vi "write_to_Sumitomo_F70.vi"(0 "VISA resource name":refnum<visa-resource-name>, 2 "Write String":string="$", 11 "error in (no error)":errorcluster) -> (4 "VISA resource name out":refnum<visa-resource-name>, 13 "Written String":string, 15 "error out":errorcluster)   [LabVIEW 2023]
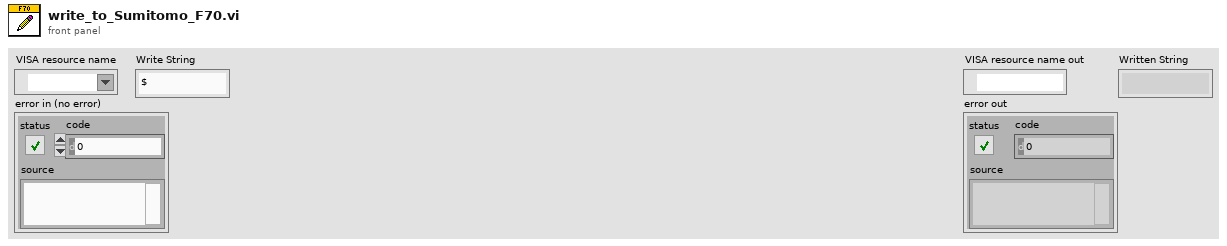
[diagram p1: front panel]
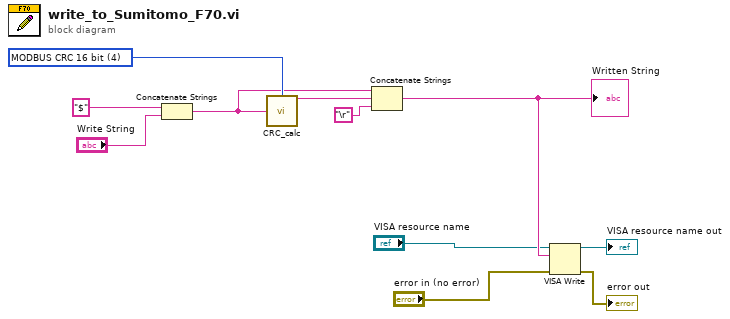
[diagram p0: block diagram]
diagram:
  w9 = u32 4 items=["XOR", "8 bit sum (MOD 100h)", "8 bit LRC", "16 bit sum (MOD 10000h)", "MODBUS CRC 16 bit", "XOR 16 bit"] ("Type (0)")
  n1 = Concatenate Strings("$", "Write String") -> (w8:string)
  n2 = call "CRC_calc.vi"("Type (0)"=w9, "String"=w8) -> ("Checksum hex"=w7:string)  [unwired: 12 in, 1 out]
  n3 = Concatenate Strings(w8, w7, "\r") -> (w5:string)
  "Written String" <- w5
  n4 = VISA Write(VISA resource name="VISA resource name", write buffer=w5, error in (no error)="error in (no error)") -> (VISA resource name out=→"VISA resource name out":refnum<visa-resource-name>, error out=→"error out":errorcluster)  [unwired: 1 out]
